vi "Add Data with TS.vi"(8 "Error In":errorcluster, 9 "Values":dbl[](array[numeric]), 10 "Time Stamp":timestamp format="%<%x %.3X>T", 11 "BNT_XtGraph in":refnum<class "BNT_XtGraph.lvclass">) -> (0 "Error Out":errorcluster, 3 "BNT_XtGraph out":refnum<class "BNT_XtGraph.lvclass">)   [LabVIEW 2019, in "BNT_XtGraph.lvlib" / "BNT_XtGraph.lvclass"]
doc: "Add actual data with one timestamp for all channels to history."
uses:
  BNT_XtGraph.lvclass
  BNT_XtGraph.lvclass/BNT_XtGraph.ctl
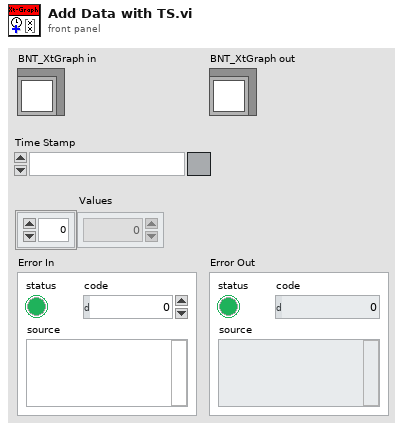
[diagram p1: front panel]
types:
  T1 = cluster{"X-t Value Pairs":cluster{"Time Stamp":timestamp, "Value":dbl}[]}[]
  T2 = cluster{"X-t Value Pairs":cluster{"Time Stamp":timestamp, "Value":dbl}[]}
  T3 = cluster{cluster{"Time Stamp":timestamp, "Value":dbl}[]}
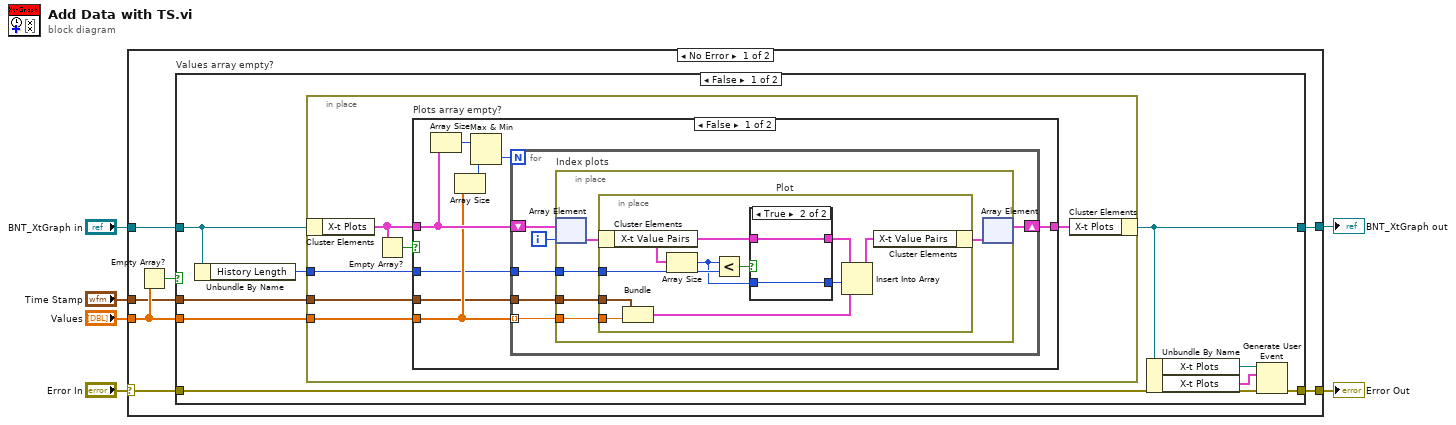
[diagram p0: block diagram]
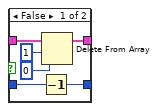
[diagram p2: hidden frame]
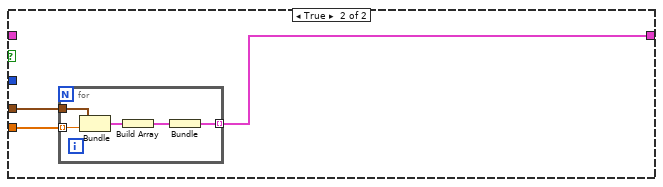
[diagram p3: hidden frame]
diagram:
  n1 = case shown="No Error" "Error In" {
    selector: "Error In" -> [w10 w77]
    tunnel: [w11 w77] -> w3
    tunnel: [w12 w76] -> w5
    tunnel: "BNT_XtGraph in" -> [w13 w76]
    tunnel: "Values" -> [w8 _]
    tunnel: "Time Stamp" -> [w7 _]
    frame No Error {
      n2 = Empty Array?(array=w8) -> (empty?=w9:bool)
      n3 = case "Values array empty?" shown="False" w9 {
        tunnel: w13 -> [w21 w75]
        tunnel: [w19 w75] -> w12
        tunnel: [w15 w74] -> w11
        tunnel: w10 -> [w16 w74]
        tunnel: w8 -> [w22 _]
        tunnel: w7 -> [w14 _]
        frame False {
          n4 = Unbundle By Name(w21) -> ("History Length"=w20:u32)
          n5 = in-place {
            in-place-border: w22 -> [w27]
            in-place-border: w20 -> [w24]
            in-place-border: w14 -> [w23]
            n6 = in-place-cluster #1(w21) -> ("X-t Plots"=w25:T1)
            n7 = Empty Array?(array=w25) -> (empty?=w28:bool)
            n8 = case "Plots array empty?" shown="False" w28 {
              tunnel: w23 -> [w29 w67]
              tunnel: w27 -> [w31 w68]
              tunnel: [w32 w66] -> w26
              tunnel: w25 -> [w33 _]
              tunnel: w24 -> [w30 _]
              frame False {
                n9 = Array Size(array=w33) -> (size(s)=w36:i32)
                n10 = Array Size(array=w31) -> (size(s)=w35:i32)
                n11 = Max & Min(x=w36, y=w35) -> (min(x,y)=w34:i32)  [unwired: 1 out]
                n12 = for {
                  N: w34 -> [_]
                  shift-right: [w40] -> w32
                  shift-left: w33 -> [w42]
                  tunnel: w31 -> [w39] mode=indexing
                  tunnel: w30 -> [w38]
                  tunnel: w29 -> [w37]
                  i -> [w41]
                  n13 = in-place "Index plots" {
                    in-place-border: w39 -> [w45]
                    in-place-border: w38 -> [w44]
                    in-place-border: w37 -> [w43]
                    n14 = in-place-array #2(w42, w41) -> (w47:T2)
                    n15 = in-place "Plot" {
                      in-place-border: w45 -> [w50]
                      in-place-border: w44 -> [w55]
                      in-place-border: w43 -> [w49]
                      n16 = in-place-cluster #3(w47) -> ("X-t Value Pairs"=w56:cluster{"Time Stamp":timestamp, "Value":dbl}[])
                      n17 = Bundle("Time Stamp"=w49, "Value"=w50) -> (w48:cluster{"Time Stamp":timestamp, "Value":dbl})  [unwired: 1 in]
                      n18 = Array Size(array=w56) -> (size(s)=w52:i32)
                      n19 = Less?(x=w52, y=w55) -> (x < y?=w57:bool)
                      n20 = case shown="True" w57 {
                        tunnel: w56 -> [w63 w65]
                        tunnel: [w62 w65] -> w54
                        tunnel: [w58 w64] -> w51
                        tunnel: w52 -> [w59 w64]
                        frame False {
                          n21 = Decrement(x=w59) -> (x-1=w58:i32)
                          n22 = Delete From Array(array=w63, length=1, index=0) -> (array with subset deleted=w62:cluster{"Time Stamp":timestamp, "Value":dbl}[])  [unwired: 1 out]
                        }
                        frame True {
                        }
                      }
                      n23 = Insert Into Array(array=w54, index=w51, new element=w48) -> (w53:cluster{"Time Stamp":timestamp, "Value":dbl}[])
                      n24 = in-place-cluster #3("X-t Value Pairs"=w53) -> (w46:T2)
                    }
                    n25 = in-place-array #2(w46) -> (w40:T1)  [unwired: 1 out]
                  }
                }
              }
              frame True {
                n26 = for {
                  tunnel: w68 -> [w72] mode=indexing
                  tunnel: w67 -> [w73]
                  tunnel: [w70] -> w66 mode=indexing
                  n27 = Bundle("Time Stamp"=w73, "Value"=w72) -> (w71:cluster{"Time Stamp":timestamp, "Value":dbl})  [unwired: 1 in]
                  n28 = Build Array(w71) -> (w69:cluster{"Time Stamp":timestamp, "Value":dbl}[])
                  n29 = Bundle(w69) -> (w70:T3)  [unwired: 1 in]
                }
              }
            }
            n30 = in-place-cluster #1("X-t Plots"=w26) -> (w19:refnum<class "BNT_XtGraph.lvclass">)
          }
          n31 = Unbundle By Name(w19) -> ("X-t Plots"=w18:refnum<user-event>, "X-t Plots"=w17:T1)
          n32 = Generate User Event(user event=w18, event data cluster=w17, error in=w16) -> (error out=w15:errorcluster)  [unwired: 1 in, 1 out]
        }
        frame True {
        }
      }
    }
    frame Error {
    }
  }
  "BNT_XtGraph out" <- w5
  "Error Out" <- w3
